vi "MCL Get Handle By Serial.vi"(11 "serial":i16) -> (3 "function return":i32)   [LabVIEW 2017, in "Madlib.lvlib"]
doc: "MADLIB_API int MCL_GetHandleBySerial(short serial);"
uses:
  Madlib.lvlib
  Madlib.dll
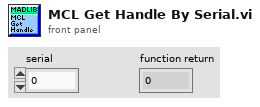
[diagram p1: front panel]
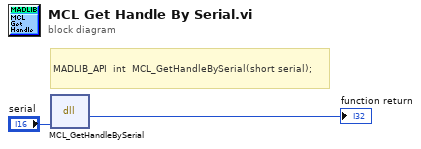
[diagram p0: block diagram]
diagram:
  # "MADLIB_API  int\t\tMCL_GetHandleBySerial(short serial);"
  n1 = dll-call lib="C:/Users/francesco/dev/pump-probe/Piezo/lvlib/Madlib.*" fn="MCL_GetHandleBySerial"("serial"="serial") -> (→"function return":i32)  [unwired: 4 in, 2 out]
